vi "video.add.vi"(6 "Series Tags":map{string, string}(c390), 8 "error in":errorcluster, 9 "Video RID":string, 10 "Datascope Name":string, 11 "asset in":refnum<class "asset.lvclass">) -> (0 "error out":errorcluster, 3 "asset out":refnum<class "asset.lvclass">)   [LabVIEW 2020, in "asset.lvclass"]
uses:
  asset.lvclass
  asset.lvclass/asset.ctl
  Nominal Client/Nominal Client.lvclass
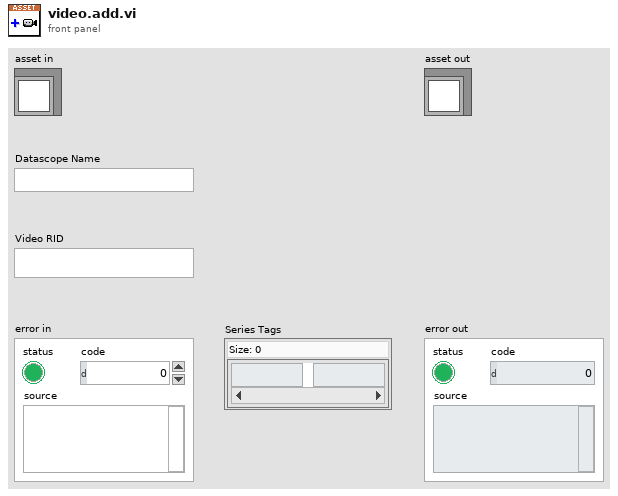
[diagram p1: front panel]
types:
  T1 = typedef "dataScopes.lvlib/links.ctl" = cluster{"URL":string, "Title":string}[]
  T2 = typedef "dataScopes.lvlib/data_scopes.ctl" = T3[]
  T3 = typedef "dataScopes.lvlib/data_scope.ctl" = cluster{"dataScopeName":string, "dataSource":T4, "seriesTags":map{string, string}, "offset":T6}
  T4 = typedef "dataScopes.lvlib/data_source.ctl" = cluster{"type":T5, "rid":string}
  T5 = typedef "dataScopes.lvlib/type.ctl" = enum16{"dataset", "connection", "logSet", "video"}
  T6 = typedef "dataScopes.lvlib/offset.ctl" = cluster{"seconds":i32, "nanos":i32, "picos":i32}
  T7 = cluster{"rid":string, "title":string, "properties":refnum<class "properties.lvclass">, "labels":refnum<class "labels.lvclass">, "Links":T1, "datascopes":T2, "createdAt":timestamp, "updatedAt":timestamp, "attachments":refnum<class "labels.lvclass">, "isStaged":bool, "isArchived":bool, "description":string, "createdBy":string, "type":string}
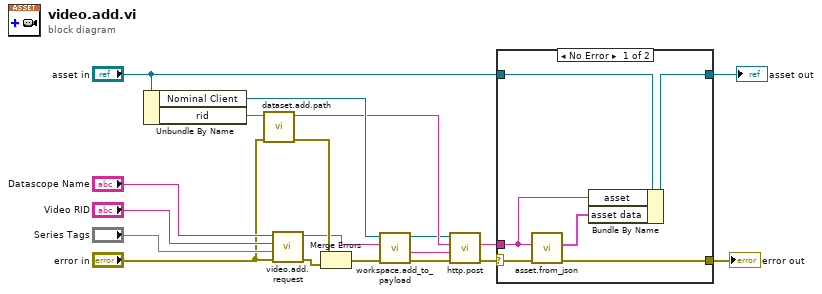
[diagram p0: block diagram]
diagram:
  n1 = Unbundle By Name("asset in") -> ("Nominal Client"=w14:refnum<class "Nominal Client.lvclass">, "rid"=w16:string)
  n2 = call "dataset.add.path.vi"("error in"="error in", "Asset RID"=w16) -> ("error out"=w15:errorcluster, "Path"=w8:string)  [unwired: 8 in]
  n3 = call "video.add.request.vi"("error in"="error in", "Series Tags"="Series Tags", "Video RID"="Video RID", "DataScope Name"="Datascope Name") -> ("error out"=w1:errorcluster, "Request"=w2:string)  [unwired: 6 in]
  n4 = Merge Errors(w15, w1) -> (w13:errorcluster)
  n5 = call "workspace.add_to_payload.vi"("error in"=w13, "JSON payload in"=w2, "Nominal Client in"=w14) -> ("error out"=w11:errorcluster, "JSON payload out"=w12:string, "Nominal Client out"=w7:refnum<class "Nominal Client.lvclass">)  [unwired: 6 in]
  n6 = call "http.post.vi"("error in"=w11, "Request body"=w12, "Path"=w8, "Nominal Client in"=w7) -> ("error out"=w10:errorcluster, "Response"=w9:string)  [unwired: 4 in, 2 out]
  n7 = case shown="No Error" w10 {
    selector: w10 -> [w25 w27]
    tunnel: [w24 w27] -> w19
    tunnel: "asset in" -> [w23 w26]
    tunnel: w9 -> [w21 _]
    tunnel: [w20 w26] -> w17
    frame No Error {
      n8 = call "asset.from_json.vi"("error in"=w25, "asset"=w21) -> ("error out"=w24:errorcluster, "Asset Data"=w22:T7)  [unwired: 8 in]
      n9 = Bundle By Name(cluster=w23, "asset"=w21, "asset data"=w22) -> (w20:refnum<class "asset.lvclass">)
    }
    frame Error {
    }
  }
  "asset out" <- w17
  "error out" <- w19
